vi "Read Boolean Text Props.vi"(8 "error in (no error)":errorcluster, 11 "Control In":refnum<vi>) -> (0 "error out":errorcluster, 2 "Boolean Text Props":T1, 3 "Control":refnum<vi>)   [LabVIEW 2020, in "VolatusGUIEditorCore.lvlib"]
uses:
  VolatusGUIEditorCore.lvlib
  Boolean Text Props.ctl
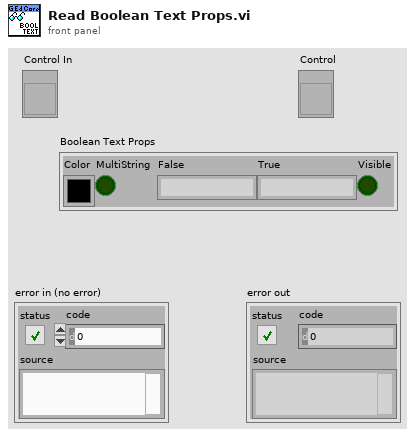
[diagram p1: front panel]
types:
  T1 = typedef "VolatusGUIEditorCore.lvlib/Boolean Text Props.ctl" = cluster{"Color":u32, "MultiString":bool, "False":string, "True":string, "Visible":bool}
  T2 = cluster{"BoolText.TextColor":u32, "MultiStrs":bool, string, string, "BoolText.Visible":bool}
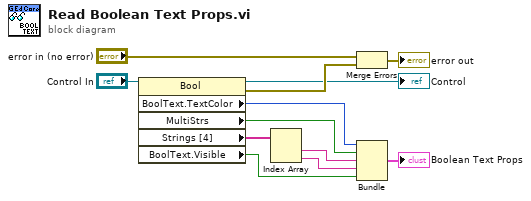
[diagram p0: block diagram]
diagram:
  n1 = property class="Bool"(reference="Control In") -> (reference out=→"Control":refnum<vi>, error out=w10:errorcluster, "BoolText.TextColor"=w6:u32, "MultiStrs"=w5:bool, "Strings [4]"=w7:string[], "BoolText.Visible"=w1:bool)  [unwired: 1 in]
  n2 = Index Array(array=w7) -> (element #1=w4:string, element #2=w3:string)  [unwired: 2 in]
  n3 = Merge Errors("error in (no error)", w10) -> (→"error out":errorcluster)
  n4 = Bundle("BoolText.TextColor"=w6, "MultiStrs"=w5, w4, w3, "BoolText.Visible"=w1) -> (→"Boolean Text Props":T2)  [unwired: 1 in]
